vi "pulser create 2d.vi"(4 "channel 0-4 energy in":u32[][](array[numeric]), 5 "labview time":dbl, 6 "pulses recieved":u32, 8 "error in (no error)":errorcluster, 11 "xy position cluster":T2) -> (0 "error out":errorcluster, 2 "live time(%)":dbl, 3 "xy position cluster out":T1, 7 "run time":dbl)   [LabVIEW 2016]
doc: "used for pulser, converts events gathered from pixie and creates a live time as well as creates the \n2d image for the pulser"
panel:
  out "sum of counts out":i32
  out "Y name output":string
  out "X name output":string
  in  "channel 0-4 energy out":u32[][](array[numeric])
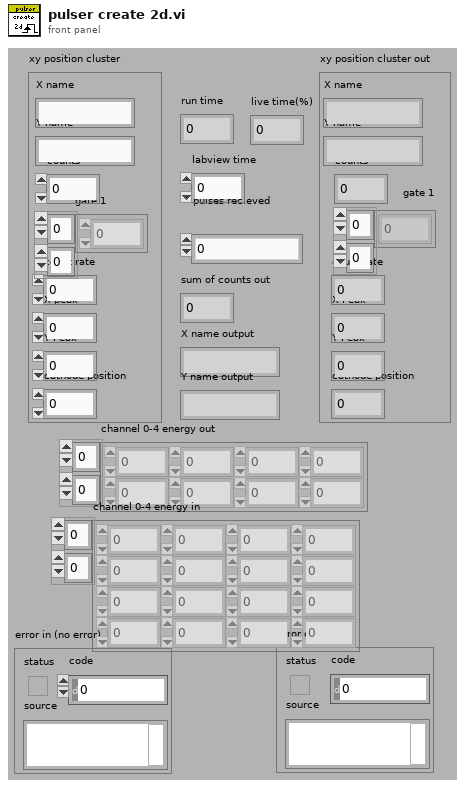
[diagram p1: front panel]
types:
  T1 = cluster{"X name":string, "Y name ":string, "counts":dbl, "gate 1":dbl[][], "count rate":dbl, "X Peak":dbl, "Y Peak":dbl, "cathode position":dbl}
  T2 = cluster{"X name":string, "Y name ":string, "counts":dbl, "gate 1":dbl[][], "count rate":dbl, "X peak":dbl, "Y Peak":dbl, "cathode position":dbl}
  T3 = typedef "energy 2d selection.ctl" = string
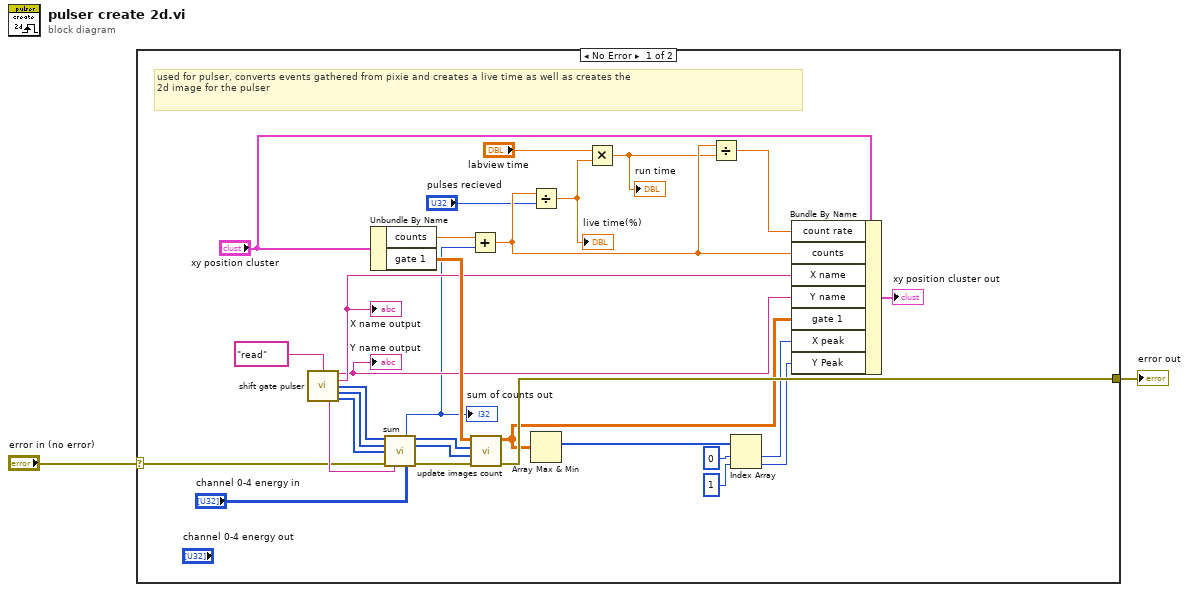
[diagram p0: block diagram]
diagram:
  n1 = case shown="No Error" "error in (no error)" {
    selector: "error in (no error)" -> [w18 w33]
    tunnel: [w17 w33] -> w1
    frame No Error {
      # "used for pulser, converts events gathered from pixie and creates a live time as well as creates the \n2d image for the pulser"
      n2 = call "shift gate pulser.vi"("shift control"="read") -> ("X name output"=w15:string, "Y name  output"=w16:string, "X range output"=w26:i32[], "Y range Max output"=w25:i32[], "Energy 2d gate out"=w24:T3, "Y range Min output"=w13:i32[])  [unwired: 8 in, 1 out]
      "Y name output" <- w15
      "X name output" <- w16
      n3 = Unbundle By Name("xy position cluster") -> ("counts"=w29:dbl, "gate 1"=w21:dbl[][])
      n4 = call "sum.vi"("X range output"=w26, "Y range Max output"=w25, "Y range Min output"=w13, "error in (no error)"=w18, "Energy 2d gate out"=w24, "Peak height  in"="channel 0-4 energy in") -> ("sum of counts out"=w12:i32, "X output array"=w20:u16[], "Y range  output"=w19:u16[], "error out"=w22:errorcluster)  [unwired: 5 in, 1 out]
      "sum of counts out" <- w12
      n5 = Add(x=w29, y=w12) -> (x+y=w32:dbl)
      n6 = call "update images count.vi"("error in (no error)"=w22, "Y axis data"=w19, "x axis data"=w20, "Image in"=w21) -> ("error out"=w17:errorcluster, "Image Out"=w8:dbl[][])  [unwired: 6 in]
      n7 = Divide(x=w32, y="pulses recieved") -> (x/y=w9:dbl)
      "live time(%)" <- w9
      n8 = Array Max & Min(array=w8) -> (max index (indices)=w7:i32[])  [unwired: 3 out]
      n9 = Multiply(x="labview time", y=w9) -> (x*y=w10:dbl)
      "run time" <- w10
      n10 = Divide(x=w32, y=w10) -> (x/y=w31:dbl)
      n11 = Index Array(array=w7, index #1=0 ("index"), index #2=1 ("index")) -> (element #1=w4:i32, element #2=w3:i32)
      n12 = Bundle By Name(cluster="xy position cluster", "count rate"=w31, "counts"=w32, "X name"=w16, "Y name"=w15, "gate 1"=w8, "X peak"=w4, "Y Peak"=w3) -> (→"xy position cluster out":T2)
    }
    frame Error {
    }
  }
  "error out" <- w1
